vi "DeQueue&VTD.vi"(0 "ModuleAdmin In":refnum<class "ModuleAdmin.lvclass">, 1 "DeQueue Type (DeQueue)":T1, 5 "timeout in ms (50)":i32=50, 11 "Error In":errorcluster, 12 "QueueArrayEntry (QMH)":T2) -> (4 "ModuleAdmin Out":refnum<class "ModuleAdmin.lvclass">, 6 "Message":string, 8 "Message Data":variant, 10 "Class":refnum<class "SensorBase.lvclass">, 14 "timed out?":bool, 15 "Error Out":errorcluster)   [LabVIEW 2018, in "SensorPlugins.lvlib"]
doc: "Dequeues the data and converts the data from the variant to the type expected by the module."
uses:
  SensorPlugins.lvlib
  SensorBaseClass/SensorBase.lvclass
  <userlib>/NIST/ModuleAdminLib/ModuleAdmin/ModuleAdmin.lvclass
  <userlib>/NIST/ModuleAdminLib/ModuleAdmin/TypeDefinitions/QueueEntry.ctl
  <userlib>/NIST/ModuleAdminLib/ModuleAdmin/TypeDefinitions/DeQueueType.ctl
  clMessage.ctl
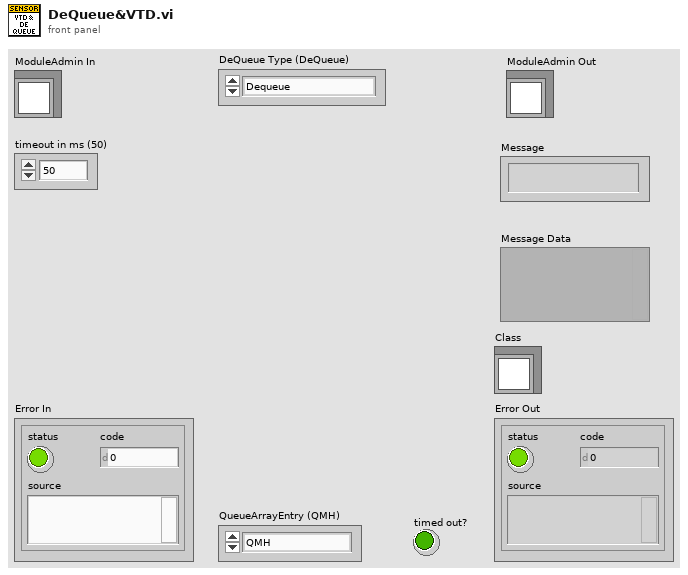
[diagram p1: front panel]
types:
  T1 = typedef "ModuleAdmin.lvlib/ModuleAdmin.lvclass/DeQueueType.ctl" = enum16{"Dequeue", "PreviewQueue"}
  T2 = typedef "ModuleAdmin.lvlib/ModuleAdmin.lvclass/QueueEntry.ctl" = enum16{"QMH", "Class Data", "Data Loop", "Queue 4", "Queue 5", "Queue 6", "Queue 7", "Queue 8", "Queue 9", "Queue 10"}
  T3 = typedef "SensorPlugins.lvlib/clMessage.ctl" = cluster{"Message":string, "Message Data":variant, "Class":refnum<class "SensorBase.lvclass">}
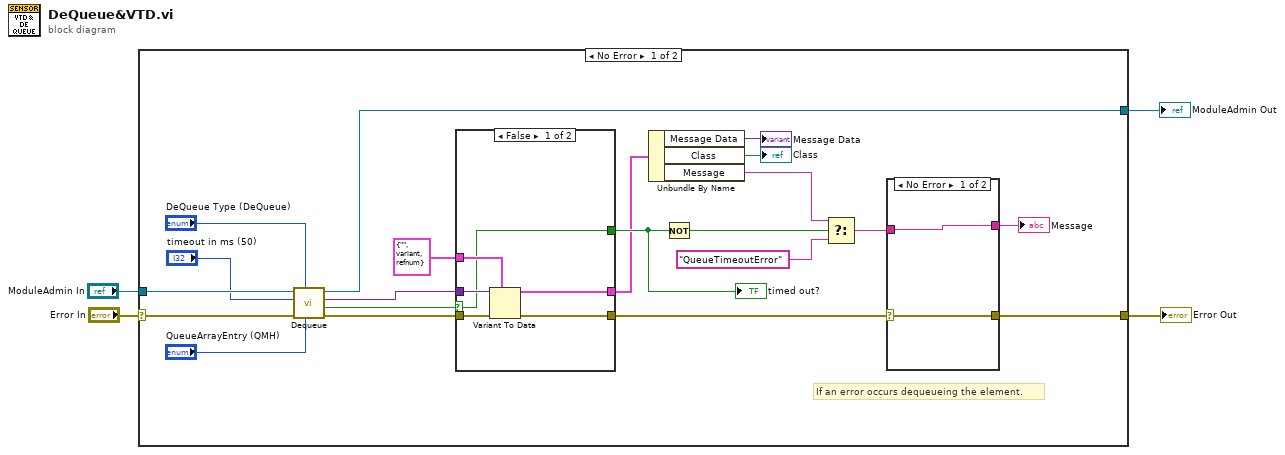
[diagram p0: block diagram]
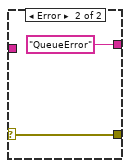
[diagram p3: hidden frame]
diagram:
  n1 = case shown="No Error" "Error In" {
    selector: "Error In" -> [w13 w40]
    tunnel: [w14 w40] -> w3
    tunnel: "ModuleAdmin In" -> [w9 w39]
    tunnel: [w6 w39] -> w1
    frame No Error {
      # "If an error occurs dequeueing the element."
      n2 = call <userlib>:"Dequeue.vi"("QueueArrayEntry (QMH)"="QueueArrayEntry (QMH)", "DeQueue Type (DeQueue)"="DeQueue Type (DeQueue)", "error in (no error)"=w13, "timeout in ms (100)"="timeout in ms (50)", "ModuleAdmin In"=w9) -> ("error out"=w12:errorcluster, "timed out?"=w10:bool, "Element"=w11:variant, "ModuleAdmin Out"=w6:refnum<class "ModuleAdmin.lvclass">)  [unwired: 3 in]
      n3 = case shown="False" w10 {
        selector: w10 -> [w26 w32]
        tunnel: [w26 w32] -> w18
        tunnel: w11 -> [w31 _]
        tunnel: w12 -> [w30 w34]
        tunnel: [w29 w34] -> w17
        tunnel: [w28 w33] -> w15
        tunnel: T3 {"Message"="", "Message Data"=variant, "Class"=refnum} ("clMessage") -> [w27 w33]
        frame False {
          n4 = Variant To Data(error in=w30, type=w27, Variant=w31) -> (data=w28:T3, error out=w29:errorcluster)
        }
        frame True {
          # "If the queue timeout \ndon't attempt to convert\nthe variant data\nsince there will be no data"
        }
      }
      "timed out?" <- w18
      n5 = Unbundle By Name(w15) -> ("Message Data"=→"Message Data":variant, "Class"=→"Class":refnum<class "SensorBase.lvclass">, "Message"=w22:string)
      n6 = Not(x=w18) -> (.not. x?=w21:bool)
      n7 = Select(t=w22, s=w21, f="QueueTimeoutError" ("Message")) -> (s? t:f=w20:string)
      n8 = case shown="No Error" w17 {
        selector: w17 -> [w35 w37]
        tunnel: w20 -> [w36 _]
        tunnel: [w36 "QueueError" ("Message")] -> w23
        tunnel: [w35 w37] -> w14
        frame No Error {
        }
        frame Error {
        }
      }
      "Message" <- w23
    }
    frame Error {
    }
  }
  "Error Out" <- w3
  "ModuleAdmin Out" <- w1
